vi "AlazarSampling - ATS-SDK.vi"(8 "error in (no error)":errorcluster, 9 "Time Out (s)":dbl, 10 "Sampling (Hz)":dbl, 11 "Handle":u32) -> (0 "error out":errorcluster, 1 "Return Code":u32, 3 "Handle Out":u32)   [LabVIEW 2022 SP3]
doc: "_____AlazarTech, Scope_____\n\nConfigure the capture clock circuitry."
panel:
  in  "Numeric":i32 format="%x"
  out "Array":dbl[](array[numeric])
  in  "Sample Rate Constant":u32(ring)=48 items=["1 kS/s"=1, "2 kS/s"=2, "5 kS/s"=4, "10 kS/s"=8, "20 kS/s"=10, "50 kS/s"=12, "100 kS/s"=14, "200 kS/s"=16, "500 kS/s"=18, "1 MS/s"=20, "2 MS/s"=24, "5 MS/s"=26, "10 MS/s"=28, "20 MS/s"=30, "25 MS/s"=33, "50 MS/s"=34, "100 MS/s"=36, "125 MS/s"=37, "160 MS/s"=38, "180 MS/s"=39, "200 MS/s"=40, "250 MS/s"=43, "500 MS/s"=48, "800 MS/s"=50, "1000 MS/s"=53, "1200 MS/s"=55, "1500 MS/s"=58, "1800 MS/s"=61, "2000 MS/s"=63, "2400 MS/s"=106, "3000 MS/s"=117, "3600 MS/s"=123, "4000 MS/s"=128]
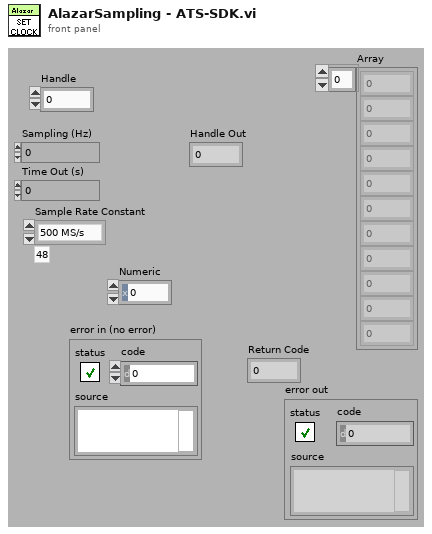
[diagram p1: front panel]
types:
  T1 = typedef "LVStringsAndValuesArrayTypeDef_U32.ctl" = cluster{"String":string, "Value":u32}[]
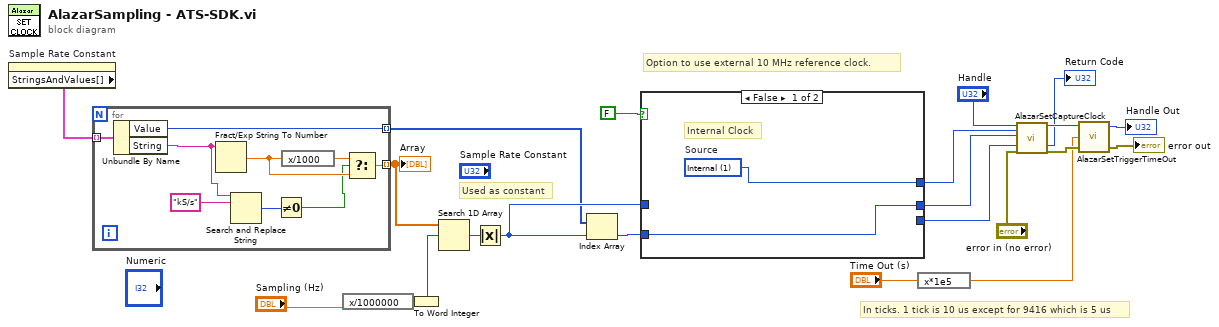
[diagram p0: block diagram]
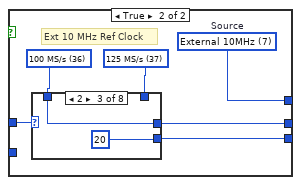
[diagram p2: hidden frame]
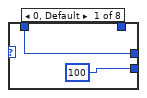
[diagram p3: hidden frame]
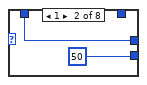
[diagram p4: hidden frame]
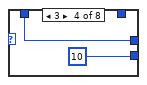
[diagram p5: hidden frame]
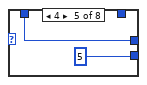
[diagram p6: hidden frame]
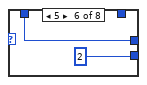
[diagram p7: hidden frame]
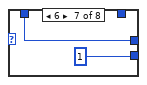
[diagram p8: hidden frame]
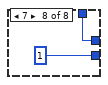
[diagram p9: hidden frame]
diagram:
  # "In ticks. 1 tick is 10 us except for 9416 which is 5 us"
  # "Used as constant"
  # "Option to use external 10 MHz reference clock."
  n1 = property on="Sample Rate Constant" class="Ring (strict)"() -> ("StringsAndValues[]"=w5:T1)  [unwired: 2 in, 2 out]
  n2 = for {
    tunnel: w5 -> [w31] mode=indexing
    tunnel: [w30] -> w4 mode=indexing
    tunnel: [w23] -> w3 mode=indexing
    n3 = Unbundle By Name(w31) -> ("Value"=w30:u32, "String"=w27:string)
    n4 = Fract/Exp String To Number(string=w27) -> (number=w28:dbl)  [unwired: 3 in, 1 out]
    n5 = Search and Replace String(input string=w27, search string="kS/s" ("format string")) -> (number of replacements=w24:i32)  [unwired: 6 in, 3 out]
    n6 = Not Equal To 0?(x=w24) -> (x != 0?=w26:bool)
    n7 = expression code="x/1000"(w28) -> (w29:dbl)
    n8 = Select(t=w29, s=w26, f=w28) -> (s? t:f=w23:dbl)
  }
  "Array" <- w3
  n9 = expression code="x/1000000"("Sampling (Hz)") -> (w22:dbl)
  n10 = To Word Integer(number=w22) -> (16bit integer=w1:i16)
  n11 = Search 1D Array(1D array=w3, element=w1) -> (index of element=w21:i32)  [unwired: 1 in]
  n12 = Absolute Value(x=w21) -> (abs(x)=w16:i32)
  n13 = Index Array(array=w4, index=w16) -> (element=w18:u32)
  n14 = case shown="False" FALSE {
    tunnel: [w33 w36] -> w14
    tunnel: w18 -> [w32 _]
    tunnel: [w32 w38] -> w11
    tunnel: w16 -> [_ w39]
    tunnel: [_ w37] -> w13
    frame False {
      w33 = u32 1 items=["Internal"=1, "Fast External"=2, "Medium External"=3, "Slow External"=4, "External AC"=5, "External DC"=6, "External 10MHz"=7]  # Source
      # "Internal Clock"
    }
    frame True {
      w34 = u32 37 items=["1 kS/s"=1, "2 kS/s"=2, "5 kS/s"=4, "10 kS/s"=8, "20 kS/s"=10, "50 kS/s"=12, "100 kS/s"=14, "200 kS/s"=16, "500 kS/s"=18, "1 MS/s"=20, "2 MS/s"=24, "5 MS/s"=26, "10 MS/s"=28, "20 MS/s"=30, "25 MS/s"=33, "50 MS/s"=34, "100 MS/s"=36, "125 MS/s"=37, "160 MS/s"=38, "180 MS/s"=39, "250 MS/s"=43, "500 MS/s"=48, "800 MS/s"=50, "1000 MS/s"=53, "1200 MS/s"=55, "1500 MS/s"=58, "1800 MS/s"=61] ("Sample Rate")
      w35 = u32 36 items=["1 kS/s"=1, "2 kS/s"=2, "5 kS/s"=4, "10 kS/s"=8, "20 kS/s"=10, "50 kS/s"=12, "100 kS/s"=14, "200 kS/s"=16, "500 kS/s"=18, "1 MS/s"=20, "2 MS/s"=24, "5 MS/s"=26, "10 MS/s"=28, "20 MS/s"=30, "25 MS/s"=33, "50 MS/s"=34, "100 MS/s"=36, "125 MS/s"=37, "160 MS/s"=38, "180 MS/s"=39, "250 MS/s"=43, "500 MS/s"=48, "800 MS/s"=50, "1000 MS/s"=53, "1200 MS/s"=55, "1500 MS/s"=58, "1800 MS/s"=61] ("Sample Rate")
      w36 = u32 7 items=["Internal"=1, "Fast External"=2, "Medium External"=3, "Slow External"=4, "External AC"=5, "External DC"=6, "External 10MHz"=7]  # Source
      # "Ext 10 MHz Ref Clock"
      n15 = case shown="2" w39 {
        tunnel: [w41 w43 w45 w47 w49 w51 w53 w55] -> w38
        tunnel: w34 -> [_ _ _ _ _ _ _ w55]
        tunnel: [u32 100 ("Source") u32 50 ("Source") u32 20 ("Source") u32 10 ("Source") u32 5 ("Source") u32 2 ("Source") u32 1 ("Source") u32 1 ("Source")] -> w37
        tunnel: w35 -> [w41 w43 w45 w47 w49 w51 w53 _]
        frame 0, Default {
        }
        frame 1 {
        }
        frame 2 {
        }
        frame 3 {
        }
        frame 4 {
        }
        frame 5 {
        }
        frame 6 {
        }
        frame 7 {
        }
      }
    }
  }
  n16 = expression code="x*1e5"("Time Out (s)") -> (w2:dbl)
  n17 = call "AlazarSetCaptureClock.vi"("Handle"="Handle", "Source"=w14, "Sample Rate"=w11, "Decimation"=w13, "error in (no error)"="error in (no error)") -> ("Handle"=w10:u64, "Return Code"=→"Return Code":u32, "error out"=w6:errorcluster)  [unwired: 12 in]
  n18 = call "AlazarSetTriggerTimeOut.vi"("error in (no error)"=w6, "Timeout Ticks"=w2, "Handle"=w10) -> ("error out"=→"error out":errorcluster, "Handle"=→"Handle Out":u64)  [unwired: 1 out]
